vi "get_camera_framerate.vi"(8 "error in":errorcluster) -> (0 "error out":errorcluster, 1 "Camera Frame Rate":dbl, 2 "Y Resolution":i32, 3 "X Resolution":i32)   [LabVIEW 2019]
uses:
  <vilib>/vision/driver/IMAQdx.llb/IMAQdx Acquisition Mode.ctl
  <vilib>/vision/driver/IMAQdx.llb/IMAQdx Buffer Number Mode.ctl
  ParametersGlobal.vi
  <vilib>/vision/driver/NI_Vision_Acquisition_Software.lvlib
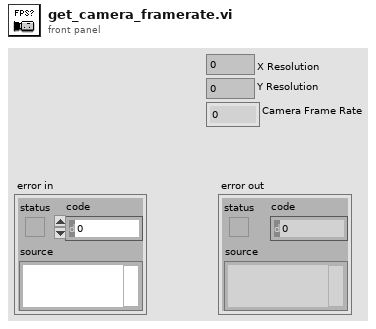
[diagram p1: front panel]
types:
  T1 = typedef "NI_Vision_Acquisition_Software.lvlib/IMAQdx Acquisition Mode.ctl" = enum32{"One Shot", "Continuous"}
  T2 = typedef "Image Type" = u32
  T3 = typedef "IMAQdx.ctl" = refnum<k21>
  T4 = typedef "IMAQ Image.ctl" = refnum<image>
  T5 = typedef "NI_Vision_Acquisition_Software.lvlib/IMAQdx Buffer Number Mode.ctl" = enum32{"Next", "Last", "Buffer Number", "Every", "Last New"}
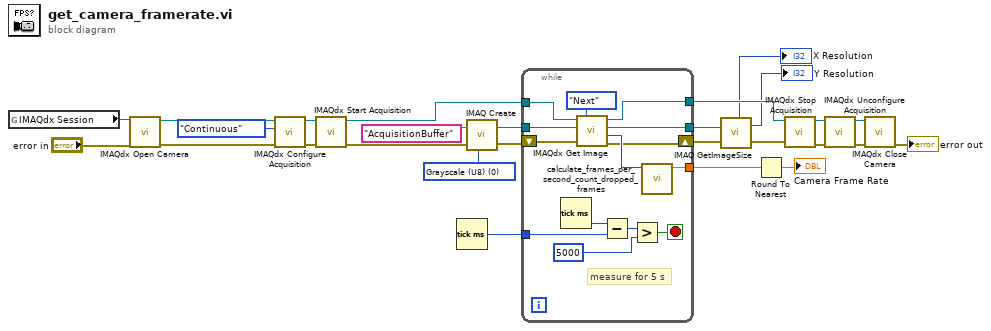
[diagram p0: block diagram]
diagram:
  w10 = T2 0 items=["Grayscale (U8)", "Grayscale (I16)", "Grayscale (SGL)", "Complex (CSG)", "RGB (U32)", "HSL (U32)", "RGB (U64)"] ("Image Type")
  n1 = global read "ParametersGlobal.vi" "IMAQdx Session"() -> (w27:T3)
  n2 = call <vilib>:"IMAQdx Open Camera.vi"("error in"="error in", "Session In"=w27) -> ("error out"=w17:errorcluster, "Session Out"=w16:T3)  [unwired: 8 in]
  n3 = call <vilib>:"IMAQdx Configure Acquisition.vi"("error in"=w17, "Continuous?"=IMAQdx_Acquisition_Mode."Continuous", "Session In"=w16) -> ("error out"=w18:errorcluster, "Session Out"=w19:T3)  [unwired: 7 in]
  n4 = call <vilib>:"IMAQdx Start Acquisition.vi"("error in"=w18, "Session In"=w19) -> ("error out"=w9:errorcluster, "Session Out"=w24:T3)  [unwired: 8 in]
  n5 = Tick Count (ms)() -> (millisecond timer value=w1:u32)
  n6 = call "IMAQ Create"("Image Name"="AcquisitionBuffer", "Image Type"=w10, "error in (no error)"=w9) -> ("New Image"=w7:T4, "error out"=w8:errorcluster)  [unwired: 2 in]
  n7 = while {
    tunnel: w24 -> [w40]
    tunnel: [w34] -> w25
    shift-right: [w37] -> w13
    shift-left: w8 -> [w39]
    tunnel: [w36] -> w26
    tunnel: [w35] -> w5
    tunnel: w7 -> [w33]
    tunnel: w1 -> [w32]
    stop <- w28 stop-if-true
    # "measure for 5 s"
    n8 = Tick Count (ms)() -> (millisecond timer value=w31:u32)
    n9 = call <vilib>:"IMAQdx Get Image.vi"("Buffer Number Mode (Next)"=IMAQdx_Buffer_Number_Mode."Next", "error in"=w39, "Image In"=w33, "Session In"=w40) -> ("error out"=w37:errorcluster, "Buffer Number Out"=w38:u32, "Image Out"=w35:T4, "Session Out"=w34:T3)  [unwired: 4 in]
    n10 = Subtract(x=w31, y=w32) -> (x-y=w30:u32)
    n11 = Greater?(x=w30, y=u32 5000) -> (0:w28:bool)
    n12 = call "calculate_frames_per_second_count_dropped_frames.vi"("Buffer Number"=w38) -> ("Acquired Frames/s"=w36:dbl)  [unwired: 8 in, 2 out]
  }
  n13 = call "IMAQ GetImageSize"("Image"=w5, "error in (no error)"=w13) -> ("Y Resolution"=→"Y Resolution":i32, "X Resolution"=→"X Resolution":i32, "error out"=w12:errorcluster)  [unwired: 2 in]
  n14 = Round To Nearest(number=w26) -> (nearest integer value=→"Camera Frame Rate":dbl)
  n15 = call <vilib>:"IMAQdx Stop Acquisition.vi"("error in"=w12, "Session In"=w25) -> ("error out"=w23:errorcluster, "Session Out"=w22:T3)  [unwired: 8 in]
  n16 = call <vilib>:"IMAQdx Unconfigure Acquisition.vi"("error in"=w23, "Session In"=w22) -> ("error out"=w20:errorcluster, "Session Out"=w21:T3)  [unwired: 8 in]
  n17 = call <vilib>:"IMAQdx Close Camera.vi"("error in"=w20, "Session In"=w21) -> ("error out"=→"error out":errorcluster)  [unwired: 9 in]
